vi "Analog_Input_1.vi"() -> ()   [LabVIEW 2019]
uses:
  <vilib>/DAQmx/read.llb/DAQmx Read (Analog 1D Wfm NChan NSamp).vi
  <vilib>/DAQmx/create/channels.llb/DAQmx Create Channel (AI-Voltage-Basic).vi
  <vilib>/DAQmx/configure/trigger.llb/DAQmx Start Trigger (Digital Edge).vi
  <vilib>/DAQmx/configure/timing.llb/DAQmx Timing (Sample Clock).vi
  <vilib>/DAQmx/miscellaneous.llb/DAQmx Fill In Error Info.vi
panel:
  in  "minimum value":dbl=-5.0 caption="최소값" format="%0.2f"
  in  "maximum value":dbl=5.0 caption="최대값" format="%0.2f"
  in  "rate":dbl=1000.0 caption="속도" format="%0.2f"
  in  "edge":i32(ring)=10280 caption="에지" items=["상승"=10280, "하강"=10171]
  in  "physical channels":tag caption="물리적 채널"
  in  "source":tag caption="소스"
  in  "정지버튼":bool
  out "웨이브폼 그래프":waveform(dbl)[](graph)
  in  "채널당 샘플 개수 (바가지 사이즈)":i32
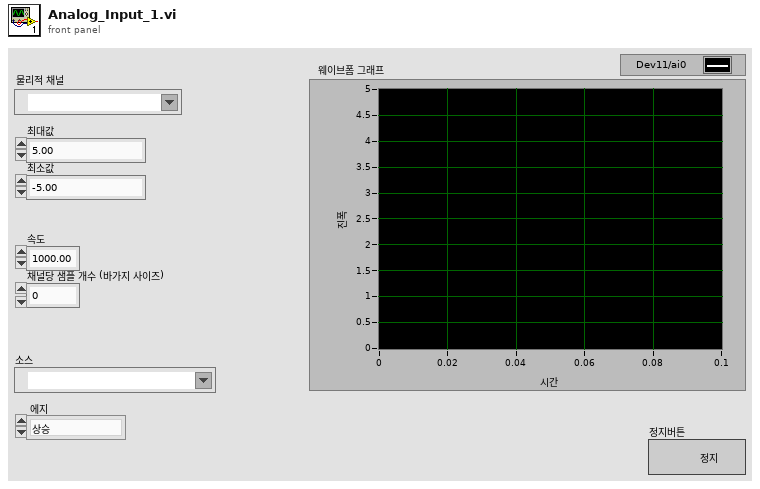
[diagram p1: front panel]
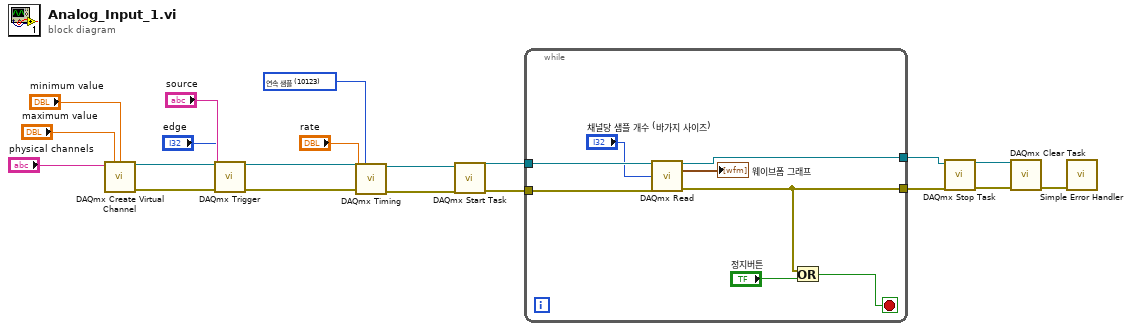
[diagram p0: block diagram]
diagram:
  w7 = 10123 items=["유한 샘플"=10178, "연속 샘플"=10123, "하드웨어 타이밍에 의한 단일 포인트"=12522] ("sample mode")
  n1 = call-poly <vilib>:"DAQmx Create Virtual Channel.vi"("maximum value"="maximum value", "minimum value"="minimum value", "physical channels"="physical channels") -> ("task out"=w20:refnum<k21>, "error out"=w19:errorcluster)  [unwired: 11 in]
  n2 = call-poly <vilib>:"DAQmx Trigger.vi"("task/channels in"=w20, "source"="source", "edge"="edge", "error in"=w19) -> ("task out"=w18:refnum<k21>, "error out"=w13:errorcluster)  [unwired: 10 in]
  n3 = call-poly <vilib>:"DAQmx Timing.vi"("task/channels in"=w18, "sample mode"=w7, "rate"="rate", "error in"=w13) -> ("task out"=w17:refnum<k21>, "error out"=w14:errorcluster)  [unwired: 10 in]
  n4 = call <vilib>:"DAQmx Start Task.vi"("task/channels in"=w17, "error in"=w14) -> ("task out"=w16:refnum<k21>, "error out"=w15:errorcluster)  [unwired: 12 in]
  n5 = while {
    tunnel: w16 -> [w28]
    tunnel: w15 -> [w27]
    tunnel: [w22] -> w12
    tunnel: [w21] -> w11
    stop <- w24 stop-if-true
    n6 = call-poly <vilib>:"DAQmx Read.vi"("task/channels in"=w28, "number of samples per channel"="채널당 샘플 개수 (바가지 사이즈)", "error in"=w27) -> ("task out"=w22:refnum<k21>, "data"=→"웨이브폼 그래프":waveform(dbl)[], "error out"=w21:errorcluster)  [unwired: 10 in]
    n7 = Or(x=w21, y="정지버튼") -> (x .or. y?=w24:bool)
  }
  n8 = call <vilib>:"DAQmx Stop Task.vi"("task/channels in"=w12, "error in"=w11) -> ("task out"=w10:refnum<k21>, "error out"=w9:errorcluster)  [unwired: 12 in]
  n9 = call <vilib>:"DAQmx Clear Task.vi"("task in"=w10, "error in"=w9) -> ("error out"=w8:errorcluster)  [unwired: 13 in]
  n10 = call <vilib>:"Simple Error Handler.vi"("error in (no error)"=w8) -> ()  [unwired: 4 in, 5 out]
